vi "Notify Identified.vi"(8 "error in (no error)":errorcluster, 11 "OBS in":refnum<class "OBS.lvclass">) -> (0 "error out":errorcluster, 3 "OBS out":refnum<class "OBS.lvclass">)   [LabVIEW 2022 SP3, in "obs-websocket-lv.lvlib" / "OBS.lvclass"]
uses:
  OBS.lvclass
  OBS.lvclass/OBS.ctl
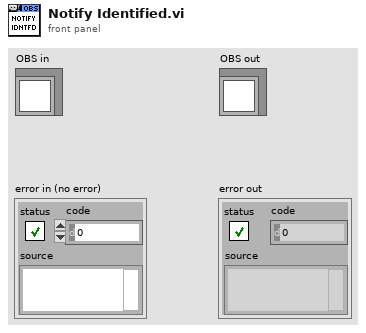
[diagram p1: front panel]
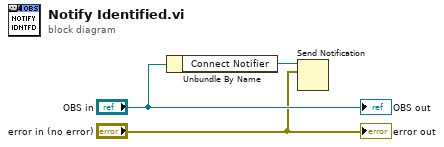
[diagram p0: block diagram]
diagram:
  n1 = Unbundle By Name("OBS in") -> ("Connect Notifier"=w2:refnum<notifier>)
  n2 = Send Notification(notification="error in (no error)", notifier=w2) -> ()  [unwired: 1 in, 2 out]
  "error out" <- "error in (no error)"
  "OBS out" <- "OBS in"
